vi "ReadWriteValveToDAQ.vi"(9 "Reactor Selector":T1(ring), 11 "DAQ Ports":bool[](array[boolean])) -> ()   [LabVIEW 2022 SP3]
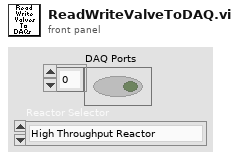
[diagram p1: front panel]
types:
  T1 = enum16{"High Throughput Reactor", "In Situ Reactor", "MLD Reactor"}
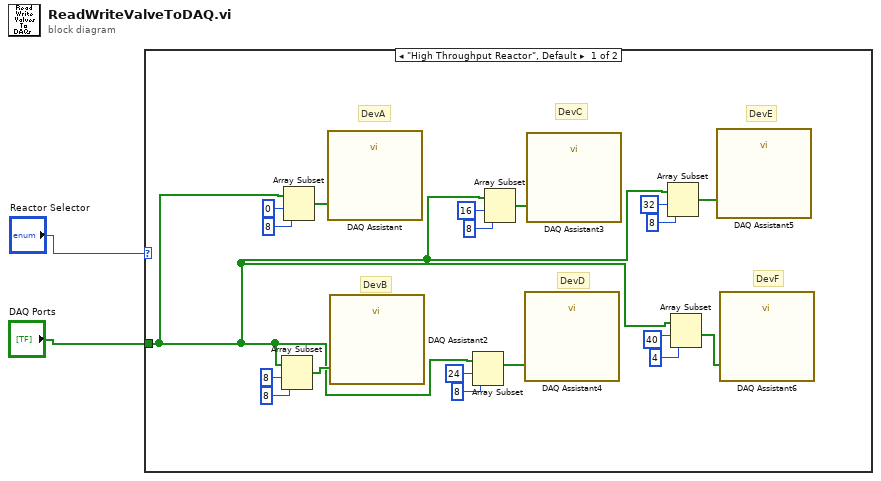
[diagram p0: block diagram]
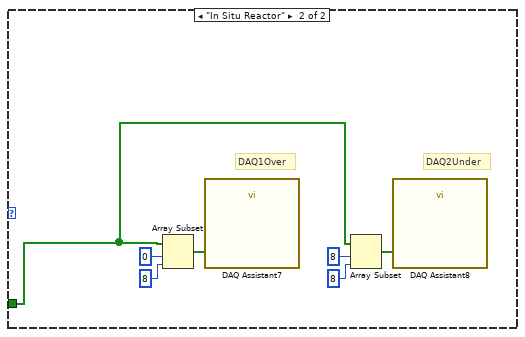
[diagram p2: hidden frame]
diagram:
  n1 = case shown="\"High Throughput Reactor\", Default" "Reactor Selector" {
    tunnel: "DAQ Ports" -> [w3 w22]
    frame "High Throughput Reactor", Default {
      # "DevF"
      # "DevE"
      # "DevC"
      # "DevD"
      # "DevB"
      # "DevA"
      n2 = Array Subset(array=w3, index=8, length=8) -> (w17:bool[])
      n3 = Array Subset(array=w3, index=0, length=8) -> (w16:bool[])
      n4 = call "DAQ Assistant"("data"=w16) -> ()  [unwired: 17 in, 2 out]
      n5 = call "DAQ Assistant2"("data"=w17) -> ()  [unwired: 17 in, 2 out]
      n6 = Array Subset(array=w3, index=24, length=8) -> (w20:bool[])
      n7 = Array Subset(array=w3, index=16, length=8) -> (w19:bool[])
      n8 = call "DAQ Assistant4"("data"=w20) -> ()  [unwired: 17 in, 2 out]
      n9 = call "DAQ Assistant3"("data"=w19) -> ()  [unwired: 17 in, 2 out]
      n10 = Array Subset(array=w3, index=32, length=8) -> (w18:bool[])
      n11 = Array Subset(array=w3, index=40, length=4) -> (w21:bool[])
      n12 = call "DAQ Assistant5"("data"=w18) -> ()  [unwired: 17 in, 2 out]
      n13 = call "DAQ Assistant6"("data"=w21) -> ()  [unwired: 17 in, 2 out]
    }
    frame "In Situ Reactor" {
      # "DAQ2Under"
      # "DAQ1Over"
      n14 = Array Subset(array=w22, index=0, length=8) -> (w28:bool[])
      n15 = call "DAQ Assistant7"("data"=w28) -> ()  [unwired: 17 in, 2 out]
      n16 = Array Subset(array=w22, index=8, length=8) -> (w23:bool[])
      n17 = call "DAQ Assistant8"("data"=w23) -> ()  [unwired: 17 in, 2 out]
    }
  }
